vi "Expose My Dependencies.vi"(8 "error in (no error)":errorcluster, 11 "SMO.SelfTerminatingOverride in":refnum<class "SMO.SelfTerminatingOverride.lvclass">) -> (0 "error out":errorcluster, 2 "[Dependencies]":refnum<class "SMO.lvclass">[](array[class]), 3 "SMO.SelfTerminatingOverride out":refnum<class "SMO.SelfTerminatingOverride.lvclass">)   [LabVIEW 2021, in "SMO.SelfTerminatingOverride.lvclass"]
uses:
  SMO.SelfTerminatingOverride.lvclass
  SMO.SelfTerminatingOverride.lvclass/SMO.SelfTerminatingOverride.ctl
  src/SMO/SMO.lvclass
  C:/Repositories/SMO/tests/_test-support-SMOs/SMO.SelfTerminating/SMO.SelfTerminating.lvclass
  C:/Repositories/SMO/src/SMO/SMO.lvclass
  C:/Repositories/SMO/tests/_test-support-SMOs/SMO.SelfTerminatingOverride/SMO.SelfTerminatingOverride.lvclass
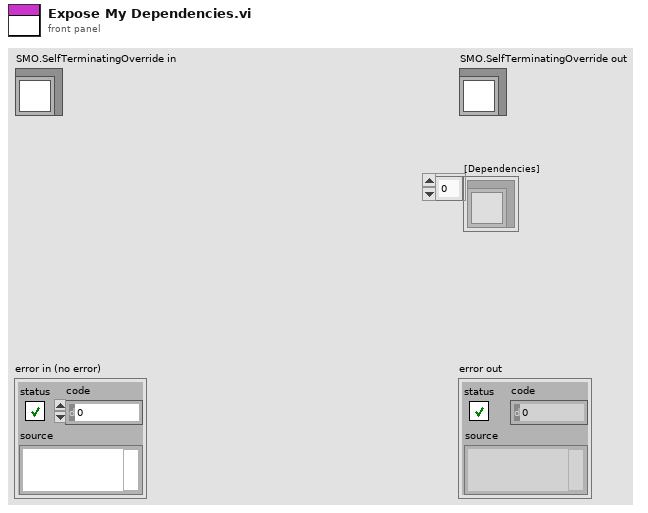
[diagram p1: front panel]
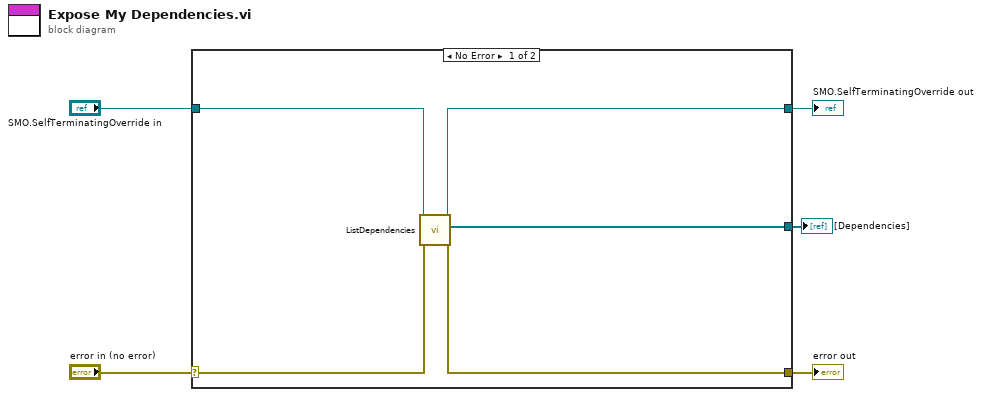
[diagram p0: block diagram]
diagram:
  n1 = case shown="No Error" "error in (no error)" {
    selector: "error in (no error)" -> [w8 w12]
    tunnel: [w7 w12] -> w4
    tunnel: [w9 w11] -> w2
    tunnel: "SMO.SelfTerminatingOverride in" -> [w10 w11]
    tunnel: [w6 _] -> w1
    frame No Error {
      n2 = call "ListDependencies.vi"("error in (no error)"=w8, "SMO in"=w10) -> ("error out"=w7:errorcluster, "[Dependencies]"=w6:refnum<class "SMO.lvclass">[], "SMO out"=w9:refnum<class "SMO.SelfTerminatingOverride.lvclass">)  [unwired: 6 in, 1 out]
    }
    frame Error {
    }
  }
  "error out" <- w4
  "SMO.SelfTerminatingOverride out" <- w2
  "[Dependencies]" <- w1
